vi "XylophonisNew.vi"() -> ()   [LabVIEW 2018]
panel:
  in  "RESET Button":bool
  out "Notes jouees":u8[](array[numeric])
  in  "stop":bool
  out "Numeric":i32
  in  "Array":bool[](array[boolean])=[FALSE, FALSE, FALSE, FALSE, FALSE, FALSE, FALSE, FALSE]
  out "Messure Musicale":dbl(graph)
  in  "File Path Control 2":path
  in  "Save Button":bool
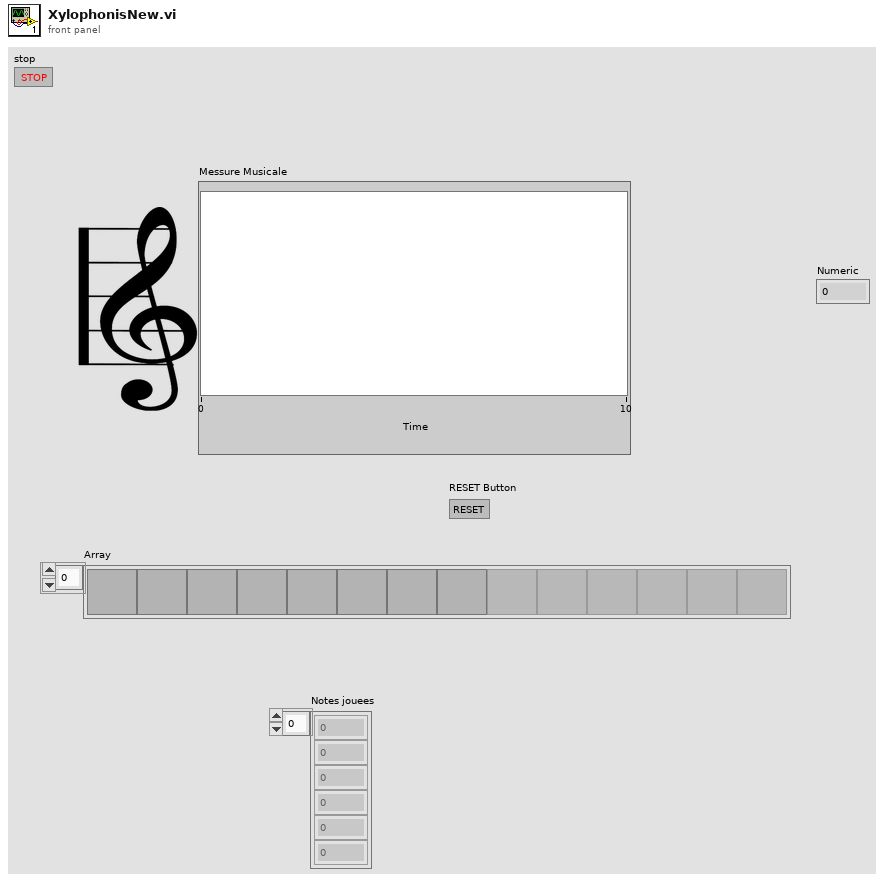
[diagram p1: front panel]
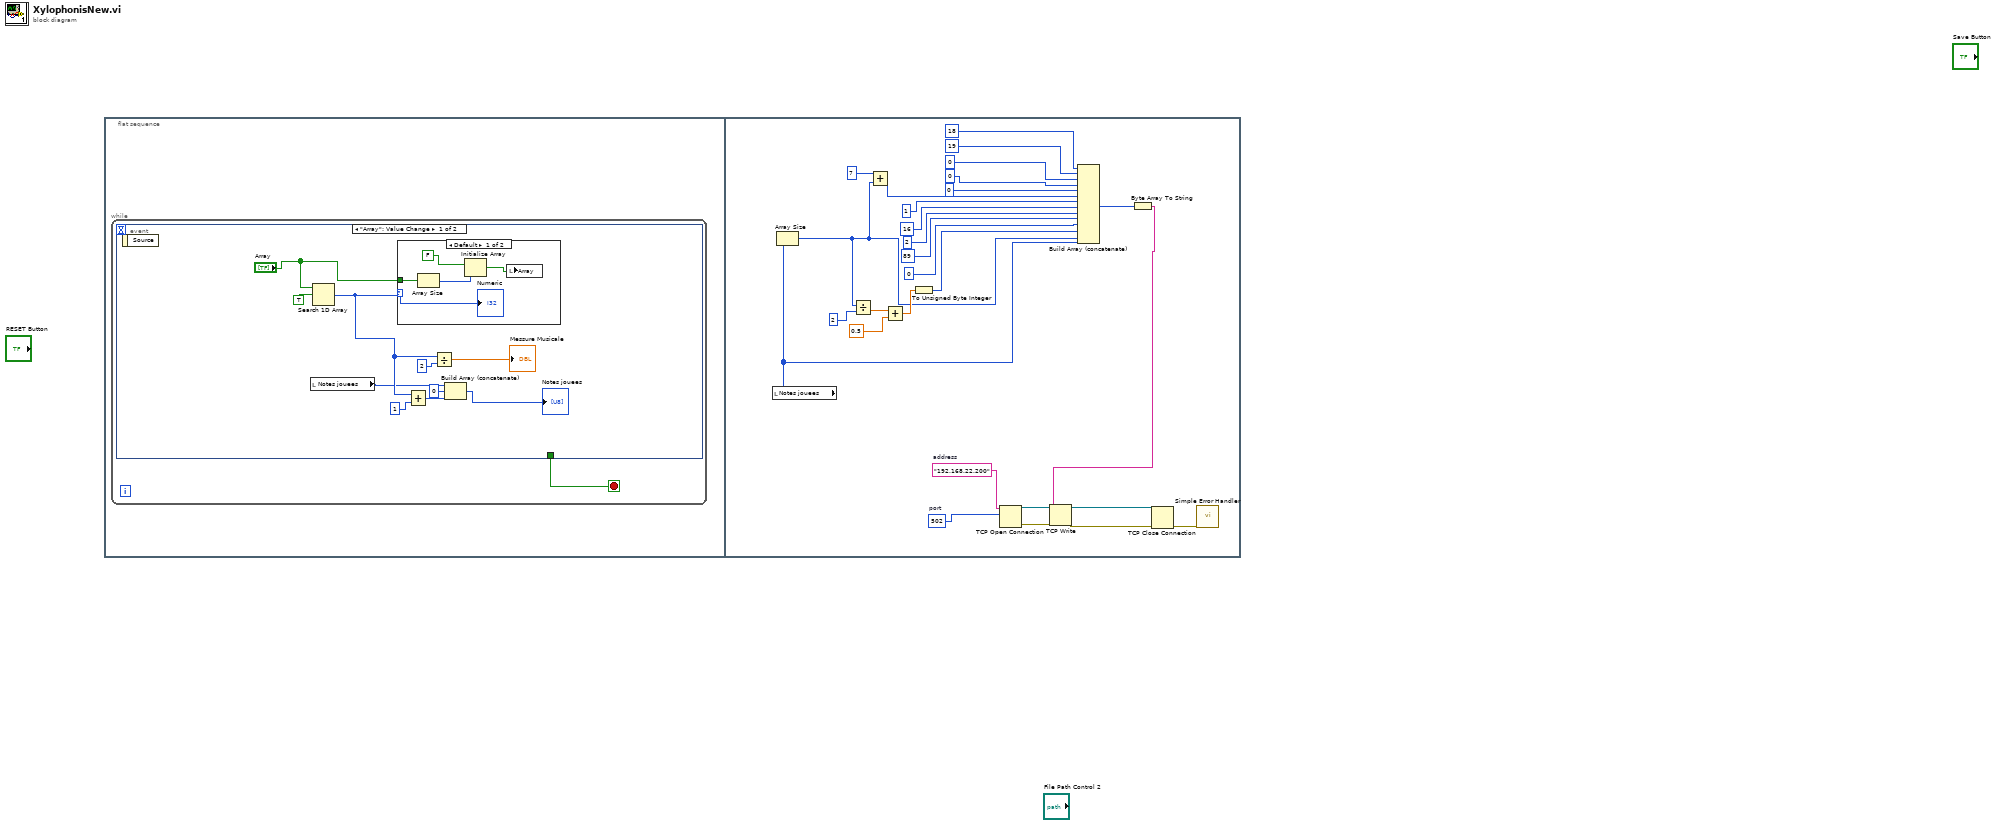
[diagram p0: block diagram]
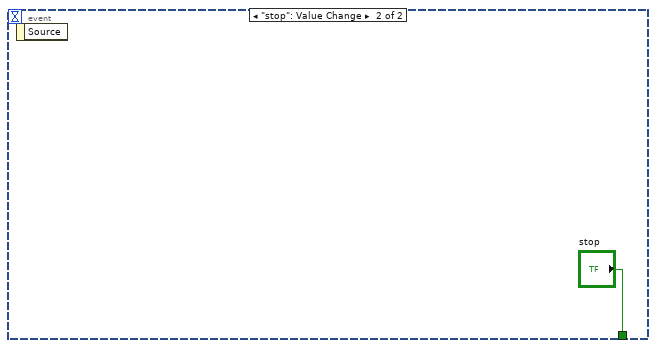
[diagram p3: hidden frame]
diagram:
  n1 = flat-sequence {
    frame #0 {
      n2 = while {
        stop <- w1 stop-if-true
        n3 = event shown="[0] \"Array\": Value Change" {
          selector: _ -> [_ _]
          dyn-events: _ -> [_ _]
          timeout: _ -> [_ _]
          tunnel: [_ "stop"] -> w1
          event "Array": Value Change {
            n4 = event-data() -> ()  [unwired: 1 in, 1 out]
            n5 = local read "Notes jouees"() -> (w5:u8[])
            n6 = Search 1D Array(1D array="Array", element=TRUE) -> (index of element=w7:i32)  [unwired: 1 in]
            n7 = case shown="Default" w7 {
              selector: w7 -> [w13 _]
              tunnel: "Array" -> [w14 _]
              frame Default {
                n8 = Array Size(array=w14) -> (size(s)=w16:i32)
                n9 = Initialize Array(FALSE ("element"), w16) -> (w12:bool[])
                n10 = local write "Array"(w12) -> ()
                "Numeric" <- w13
              }
              frame -1 {
              }
            }
            n11 = Add(x=w7, y=1) -> (x+y=w4:i32)
            n12 = Divide(x=w7, y=2 ("Numeric")) -> (x/y=→"Messure Musicale":dbl)
            n13 = Build Array (concatenate)(w5, 0 ("element"), w4) -> (→"Notes jouees":i32[])
          }
          event "stop": Value Change {
            n14 = event-data() -> ()  [unwired: 1 in, 1 out]
          }
        }
      }
    }
    frame #1 {
      w30 = "192.168.22.200"  # address
      w31 = 502  # port
      n15 = local read "Notes jouees"() -> (w22:u8[])
      n16 = Array Size(array=w22) -> (size(s)=w19:i32)
      n17 = Divide(x=w19, y=2) -> (x/y=w20:dbl)
      n18 = Add(x=7, y=w19) -> (x+y=w45:i32)
      n19 = Add(x=w20, y=0.5) -> (x+y=w28:dbl)
      n20 = To Unsigned Byte Integer(number=w28) -> (unsigned 8bit integer=w23:u8)
      n21 = TCP Open Connection(address=w30, remote port or service name=w31) -> (connection ID=w44:refnum<k5>, error out=w43:errorcluster)  [unwired: 3 in]
      n22 = Build Array (concatenate)(18, 19, 0, 0, 0, w45, 1, 16, 2, 89, 0, w23, w19, w22) -> (w40:i32[])
      n23 = Byte Array To String(unsigned byte array=w40) -> (string=w39:string)
      n24 = TCP Write(connection ID=w44, data in=w39, error in (no error)=w43) -> (connection ID out=w41:refnum<k5>, error out=w42:errorcluster)  [unwired: 1 in, 1 out]
      n25 = TCP Close Connection(connection ID=w41, error in (no error)=w42) -> (error out=w38:errorcluster)  [unwired: 1 in, 1 out]
      n26 = call <vilib>:"Simple Error Handler.vi"("error in (no error)"=w38) -> ()  [unwired: 4 in, 5 out]
    }
  }
